vi "Spectrogram_peng.vi"(4 "energy conservation?":bool=TRUE, 6 "window parameter":dbl=nan, 7 "time-freq config":T1={"force freq bins to power of 2?"=TRUE, "exclude Nyquist frequency?"=TRUE}, 8 "window info":cluster{"type":T2, "length":i32}={"type"=1, "length"=64} {"type" items=["Rectangle"=0, "Hanning"=1, "Hamming"=2, "Blackman-Harris"=3, "Exact Blackman"=4, "Blackman"=5, "Flat Top"=6, "4 Term B-Harris "=7, "7 Term B-Harris"=8, "Low Sidelobe"=9, "Blackman Nuttall"=11, "Triangle"=30, "Bartlett-Hanning"=31, "Bohman"=32, "Parzen"=33, "Welch"=34, "Kaiser"=60, "Dolph-Chebyshev"=61, "Gaussian"=62]}, 9 "time-freq sampling info":cluster{"time steps":i32, "frequency bins":i32}={"time steps"=-1, "frequency bins"=512}, 10 "Q":dbl[](array[numeric]), 11 "I":dbl[](array[numeric])) -> (0 "error":i32, 3 "STFT Spectrogram {X}":dbl[][](array[numeric]))   [LabVIEW 2015]
uses:
  <vilib>/Analysis/4window.llb/windowTd.ctl
  <vilib>/Analysis/baseanly.llb/Unit Vector (DBL).vi
  <vilib>/Analysis/2dsp.llb/Complex FFT.vi
  <vilib>/Analysis/0measdsp.llb/Scaled Time Domain Window (DBL).vi
  <vilib>/Analysis/NI_AALPro.lvlib
  <vilib>/Analysis/NI_AALBase.lvlib
  <vilib>/gmath/NI_Gmath.lvlib
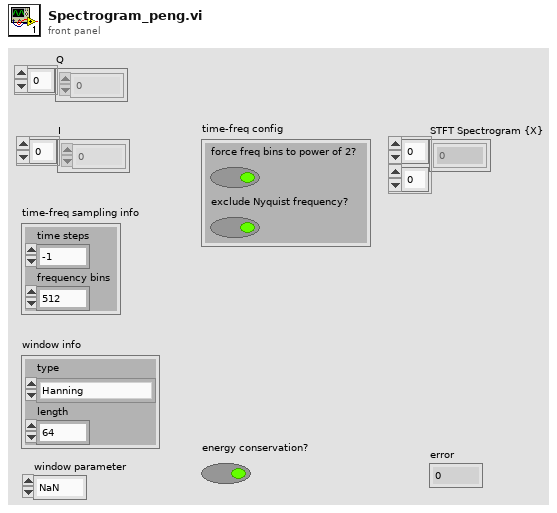
[diagram p1: front panel]
types:
  T1 = cluster{"force freq bins to power of 2?":bool, "exclude Nyquist frequency?":bool}
  T2 = typedef "NI_AALPro.lvlib/windowTd.ctl" = u32
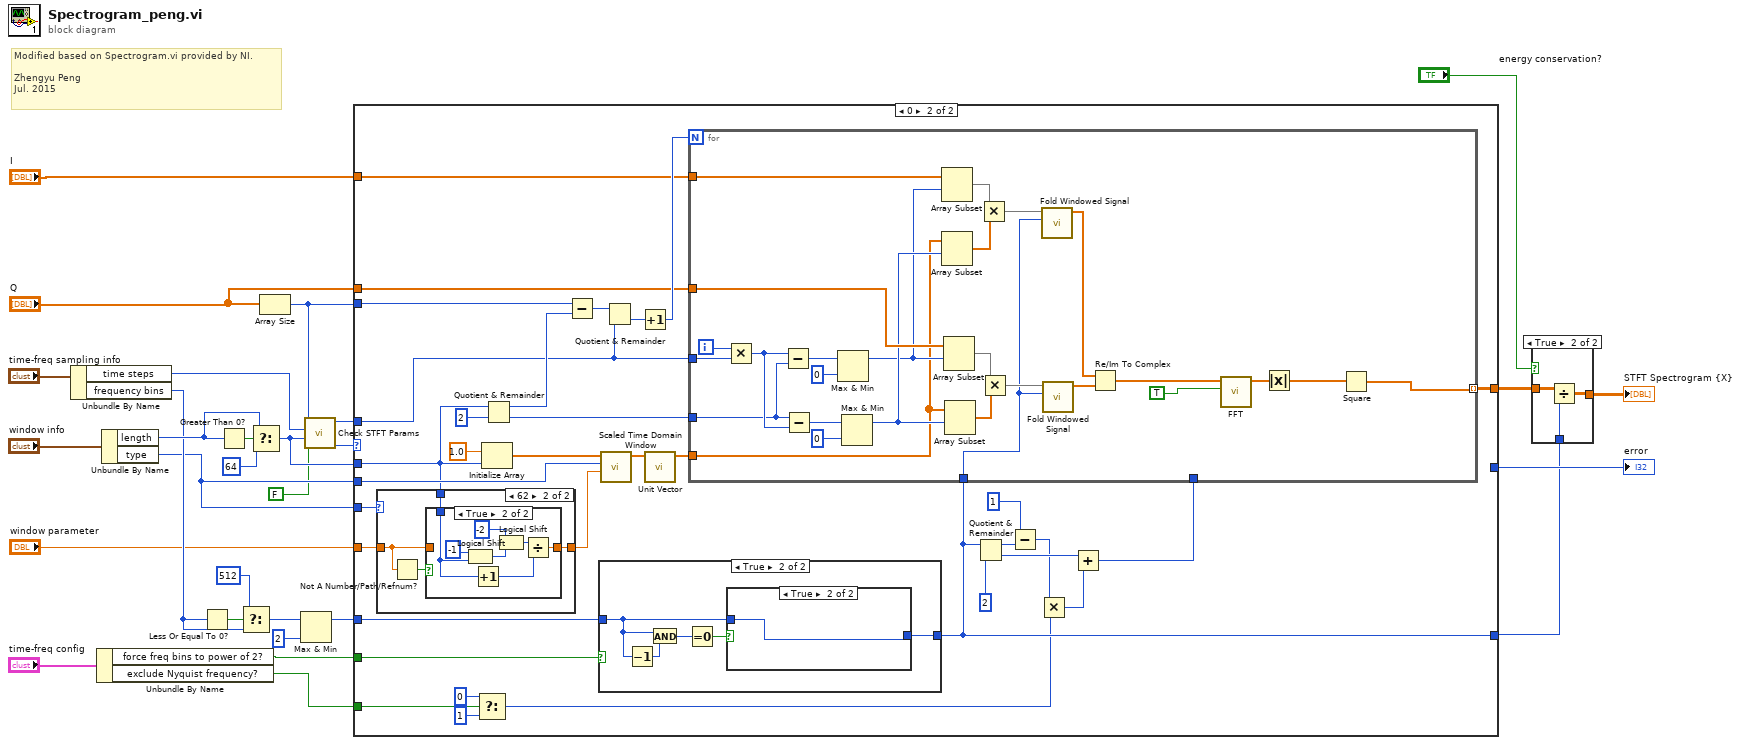
[diagram p0: block diagram]
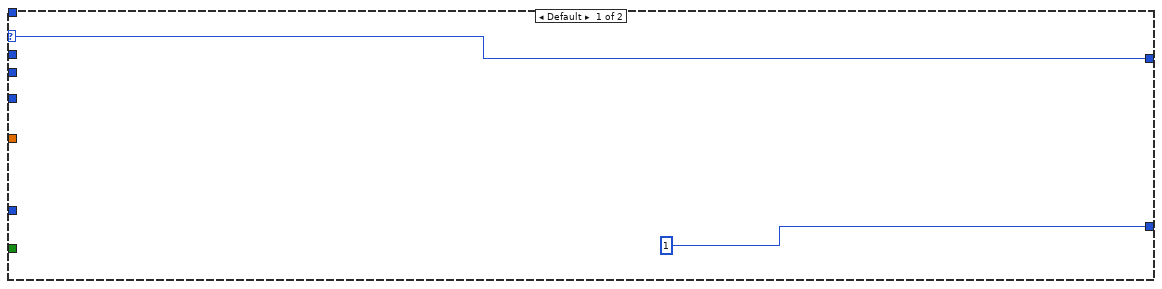
[diagram p3: hidden frame]
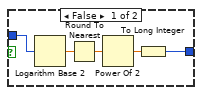
[diagram p7: hidden frame]
diagram:
  # "Modified based on Spectrogram.vi provided by NI.\n\nZhengyu Peng\nJul. 2015"
  n1 = Unbundle By Name("time-freq sampling info") -> ("time steps"=w23:i32, "frequency bins"=w11:i32)
  n2 = Unbundle By Name("time-freq config") -> ("force freq bins to power of 2?"=w18:bool, "exclude Nyquist frequency?"=w17:bool)
  n3 = Unbundle By Name("window info") -> ("length"=w21:i32, "type"=w5:T2)
  n4 = Less Or Equal To 0?(x=w11) -> (x <= 0?=w12:bool)
  n5 = Greater Than 0?(x=w21) -> (x > 0?=w26:bool)
  n6 = Select(t=512, s=w12, f=w11) -> (s? t:f=w8:i32)
  n7 = Select(t=w21, s=w26, f=64) -> (s? t:f=w10:i32)
  n8 = Array Size(array="Q") -> (size(s)=w29:i32)
  n9 = Max & Min(x=w8, y=2) -> (max(x,y)=w6:i32)  [unwired: 1 out]
  n10 = call <vilib>:"Check STFT Params.vi"("compare signal and window?"=FALSE, "windows length"=w10, "time increment"=w23, "len(X)"=w29) -> ("error"=w28:i32, "time step out"=w20:i32)  [unwired: 6 in]
  n11 = case shown="0" w28 {
    selector: w28 -> [w31 _]
    tunnel: w5 -> [_ w47]
    tunnel: "Q" -> [_ w54]
    tunnel: [_ w48] -> w15
    tunnel: w29 -> [_ w60]
    tunnel: [w31 _] -> w27
    tunnel: w20 -> [_ w57]
    tunnel: w18 -> [_ w61]
    tunnel: w17 -> [_ w51]
    tunnel: [1 ("frequency bins") w41] -> w13
    tunnel: w10 -> [_ w46]
    tunnel: w6 -> [_ w45]
    tunnel: w5 -> [_ w43]
    tunnel: "window parameter" -> [_ w33]
    tunnel: "I" -> [_ w32]
    frame Default {
    }
    frame 0 {
      n12 = case shown="62" w43 {
        tunnel: w46 -> [_ w70]
        tunnel: [w66 w69] -> w44
        tunnel: w33 -> [w66 w67]
        frame 0, Default {
        }
        frame 62 {
          n13 = Not A Number/Path/Refnum?(number/path/refnum=w67) -> (NaN/Path/Refnum?=w68:bool)
          n14 = case shown="True" w68 {
            tunnel: w70 -> [_ w74]
            tunnel: [w71 w72] -> w69
            tunnel: w67 -> [w71 _]
            frame False {
            }
            frame True {
              n15 = Logical Shift(y=-1, x=w74) -> (x << y=w77:i32)
              n16 = Increment(x=w74) -> (x+1=w73:i32)
              n17 = Logical Shift(y=-2, x=w77) -> (x << y=w78:i32)
              n18 = Divide(x=w78, y=w73) -> (x/y=w72:dbl)
            }
          }
        }
      }
      n19 = Select(t=0, s=w51, f=1) -> (s? t:f=w39:i32)
      n20 = Initialize Array(1.0 ("element"), w46) -> (w63:dbl[])
      n21 = Quotient & Remainder(x=w46, y=2) -> (x-y*floor(x/y)=w59:i32, floor(x/y)=w52:i32)
      n22 = Subtract(x=w60, y=w59) -> (x-y=w58:i32)
      n23 = case shown="True" w61 {
        tunnel: w45 -> [w106 w108]
        tunnel: [w106 w107] -> w41
        frame False {
        }
        frame True {
          n24 = Decrement(x=w108) -> (x-1=w111:i32)
          n25 = And(x=w108, y=w111) -> (x .and. y?=w110:i32)
          n26 = Equal To 0?(x=w110) -> (x = 0?=w109:bool)
          n27 = case shown="True" w109 {
            tunnel: w108 -> [w116 w117]
            tunnel: [w112 w117] -> w107
            frame False {
              n28 = Logarithm Base 2(1:w116) -> (0:w115:dbl)
              n29 = Round To Nearest(number=w115) -> (nearest integer value=w114:dbl)
              n30 = Power Of 2(x=w114) -> (2^x=w113:dbl)
              n31 = To Long Integer(number=w113) -> (32bit integer=w112:i32)
            }
            frame True {
            }
          }
        }
      }
      n32 = call-poly <vilib>:"Scaled Time Domain Window.vi"("window parameter"=w44, "window"=w47, "X"=w63) -> ("Windowed X"=w62:dbl[])  [unwired: 6 in, 2 out]
      n33 = Quotient & Remainder(x=w58, y=w57) -> (floor(x/y)=w56:i32)  [unwired: 1 out]
      n34 = Increment(x=w56) -> (x+1=w55:i32)
      n35 = call-poly <vilib>:"Unit Vector.vi"("Input Vector"=w62) -> ("Unit Vector"=w53:dbl[])  [unwired: 8 in, 2 out]
      n36 = Quotient & Remainder(x=w41, y=2) -> (x-y*floor(x/y)=w36:i32, floor(x/y)=w37:i32)
      n37 = Subtract(x=1, y=w36) -> (x-y=w34:i32)
      n38 = Multiply(x=w34, y=w39) -> (x*y=w38:i32)
      n39 = Add(x=w37, y=w38) -> (x+y=w40:i32)
      n40 = for {
        N: w55 -> [_]
        tunnel: w52 -> [w96]
        tunnel: w54 -> [w105]
        tunnel: w57 -> [w90]
        tunnel: w53 -> [w82]
        tunnel: [w98] -> w48 mode=indexing
        tunnel: w41 -> [w83]
        tunnel: w40 -> [_]
        tunnel: w32 -> [w88]
        i -> [w89]
        n41 = Multiply(x=w89, y=w90) -> (x*y=w97:i32)
        n42 = Subtract(x=w97, y=w96) -> (x-y=w94:i32)
        n43 = Subtract(x=w96, y=w97) -> (x-y=w104:i32)
        n44 = Max & Min(x=w94, y=0) -> (max(x,y)=w86:i32)  [unwired: 1 out]
        n45 = Max & Min(x=w104, y=0) -> (max(x,y)=w87:i32)  [unwired: 1 out]
        n46 = Array Subset(array=w88, index=w86) -> (w93:dbl[])  [unwired: 1 in]
        n47 = Array Subset(array=w82, index=w87) -> (w92:dbl[])  [unwired: 1 in]
        n48 = Array Subset(array=w105, index=w86) -> (w102:dbl[])  [unwired: 1 in]
        n49 = Array Subset(array=w82, index=w87) -> (w101:dbl[])  [unwired: 1 in]
        n50 = Multiply(x=w93, y=w92) -> (x*y=w91:dbl[])
        n51 = Multiply(x=w102, y=w101) -> (x*y=w100:dbl[])
        n52 = call <vilib>:"Fold Windowed Signal.vi"("frequency bins"=w83, "Windowed Signal"=w91) -> ("Folded Signal"=w85:dbl[])  [unwired: 9 in]
        n53 = call <vilib>:"Fold Windowed Signal.vi"("frequency bins"=w83, "Windowed Signal"=w100) -> ("Folded Signal"=w84:dbl[])  [unwired: 9 in]
        n54 = Re/Im To Complex(1:w84, 2:w85) -> (0:w81:cdb[])
        n55 = call-poly <vilib>:"FFT.vi"("shift?"=TRUE, "X"=w81) -> ("FFT {X}"=w99:cdb[])  [unwired: 8 in, 1 out]
        n56 = Absolute Value(x=w99) -> (abs(x)=w79:dbl[])
        n57 = Square(x=w79) -> (x^2=w98:dbl[])
      }
    }
  }
  "error" <- w27
  n58 = case shown="True" "energy conservation?" {
    tunnel: w15 -> [w118 w121]
    tunnel: w13 -> [_ w120]
    tunnel: [w118 w119] -> w14
    frame False {
    }
    frame True {
      n59 = Divide(x=w121, y=w120) -> (x/y=w119:dbl[][])
    }
  }
  "STFT Spectrogram {X}" <- w14
